vi "AODO-Create Channels (AO).vi"(0 "Tasks In":T1[](array[typedef]), 5 "Regen?":bool, 7 "Fs (Hz)":dbl, 9 "Npts":i32, 11 "error in (no error)":errorcluster) -> (4 "Tasks Out":T1[](array[typedef]), 15 "error out":errorcluster)   [LabVIEW 2020]
uses:
  Typedefs/AODO-Task Specification.ctl
  <vilib>/DAQmx/create/channels.llb/DAQmx Create Channel (AO-Voltage-Basic).vi
  <vilib>/DAQmx/configure/timing.llb/DAQmx Timing (Sample Clock).vi
  <resource>/objmgr/daqmx.rc
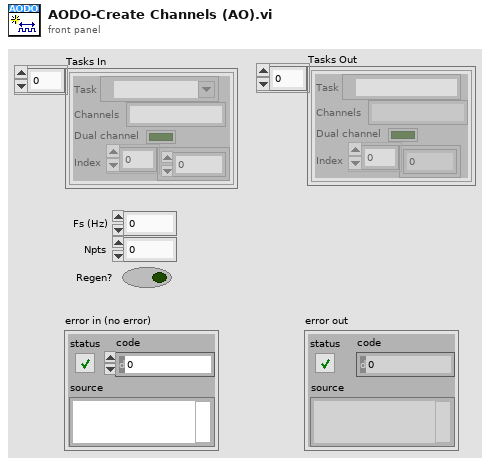
[diagram p1: front panel]
types:
  T1 = typedef "AODO-Task Specification.ctl" = cluster{"Task":refnum<k21>, "Channels":string, "Dual channel":bool, "Index":i32[]}
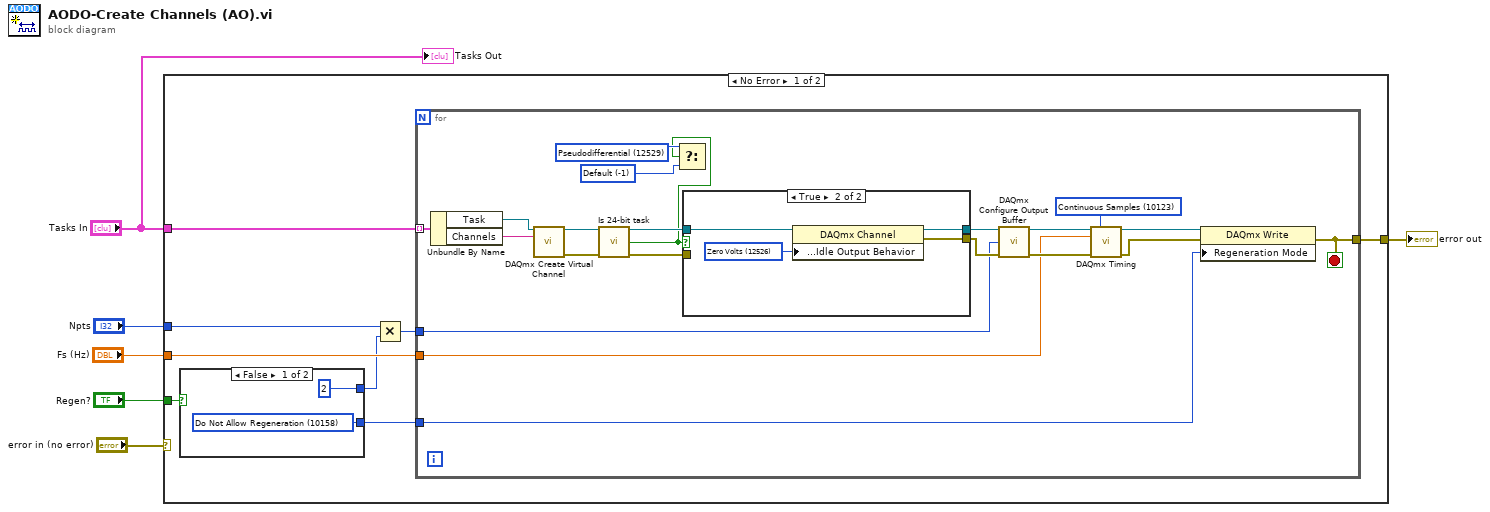
[diagram p0: block diagram]
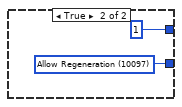
[diagram p2: hidden frame]
diagram:
  n1 = case shown="No Error" "error in (no error)" {
    selector: "error in (no error)" -> [_ w46]
    tunnel: "Tasks In" -> [w14 _]
    tunnel: "Fs (Hz)" -> [w13 _]
    tunnel: "Npts" -> [w12 _]
    tunnel: [w10 w46] -> w3
    tunnel: "Regen?" -> [w9 _]
    frame No Error {
      n2 = case shown="False" w9 {
        tunnel: [2 ("y") 1 ("y")] -> w8
        tunnel: [w15 w17] -> w7
        frame False {
          w15 = 10158 items=["Allow Regeneration"=10097, "Do Not Allow Regeneration"=10158] ("RegenMode")
        }
        frame True {
          w17 = 10097 items=["Allow Regeneration"=10097, "Do Not Allow Regeneration"=10158] ("RegenMode")
        }
      }
      n3 = Multiply(x=w12, y=w8) -> (x*y=w11:i32)
      n4 = for {
        tunnel: w14 -> [w39] mode=indexing
        tunnel: w11 -> [w20]
        tunnel: w13 -> [w28]
        tunnel: [w23] -> w10
        tunnel: w7 -> [w19]
        stop <- w23 stop-if-true
        w29 = 10123 items=["Finite Samples"=10178, "Continuous Samples"=10123, "Hardware Timed Single Point"=12522] ("sample mode")
        w34 = -1 items=["Default"=-1, "RSE"=10083, "Differential"=10106, "Pseudodifferential"=12529] ("output terminal configuration")
        w35 = 12529 items=["Default"=-1, "RSE"=10083, "Differential"=10106, "Pseudodifferential"=12529] ("output terminal configuration")
        n5 = Unbundle By Name(w39) -> ("Task"=w38:refnum<k21>, "Channels"=w21:string)
        n6 = call-poly <vilib>:"DAQmx Create Virtual Channel.vi"("task in"=w38, "physical channels"=w21) -> ("task out"=w26:refnum<k21>, "error out"=w27:errorcluster)  [unwired: 12 in]
        n7 = call "Is 24-bit task.vi"("task"=w26, "error in (no error)"=w27) -> ("task out"=w25:refnum<k21>, "is 24bit?"=w22:bool, "error out"=w24:errorcluster)  [unwired: 8 in, 3 out]
        n8 = Select(t=w35, s=w22, f=w34) -> ()  [unwired: 1 out]
        n9 = case shown="True" w22 {
          tunnel: [w41 w45] -> w37
          tunnel: [w40 w44] -> w36
          tunnel: w25 -> [w41 w42]
          tunnel: w24 -> [w40 _]
          frame False {
          }
          frame True {
            w43 = 12526 items=["Zero Volts"=12526, "High Impedance"=12527, "Maintain Existing Value"=12528] ("AO.IdleOutputBehavior")
            n10 = property class="DAQmx Channel"(reference=w42, "Analog Output:General Properties:Output Configuration:Idle Output Behavior"=w43) -> (reference out=w45:refnum<k21>, error out=w44:errorcluster)  [unwired: 1 in]
          }
        }
        n11 = call <vilib>:"DAQmx Configure Output Buffer.vi"("task/channels in"=w37, "buffer size (in samples per channel)"=w20, "error in"=w36) -> ("task out"=w31:refnum<k21>, "error out"=w30:errorcluster)  [unwired: 11 in]
        n12 = call-poly <vilib>:"DAQmx Timing.vi"("task/channels in"=w31, "sample mode"=w29, "rate"=w28, "error in"=w30) -> ("task out"=w33:refnum<k21>, "error out"=w32:errorcluster)  [unwired: 10 in]
        n13 = property class="DAQmx Write"(reference=w33, error in=w32, "Regeneration Mode"=w19) -> (error out=w23:errorcluster)  [unwired: 1 out]
      }
    }
    frame Error {
    }
  }
  "error out" <- w3
  "Tasks Out" <- "Tasks In"
